vi "TEMPLATE_Regular_Return.vi"(8 "Error In":errorcluster, 11 "LQSerialData In":refnum<class "LQSerialData.lvclass">) -> (0 "Error Out":errorcluster, 2 "Value":string, 3 "LQSerialData Out":refnum<class "LQSerialData.lvclass">)   [LabVIEW 2013, in "Template.lvlib" / "LQSerialData.lvclass"]
uses:
  LQSerialData.lvclass
  LQSerialData.lvclass/LQSerialData.ctl
  LQWidgetEngine/LQWidgetEngine.lvclass
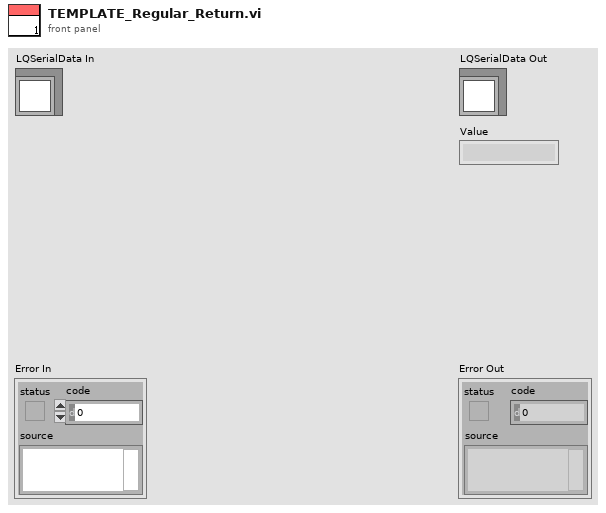
[diagram p1: front panel]
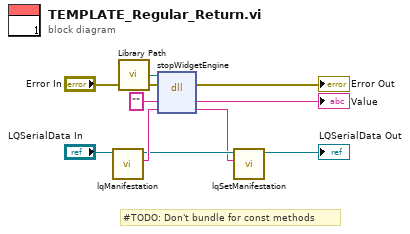
[diagram p0: block diagram]
diagram:
  # "#TODO: Don't bundle for const methods"
  n1 = call "lqManifestation.vi"("LQSerialData in"="LQSerialData In") -> ("Manifestation"=w6:string, "LQSerialData out"=w4:refnum<class "LQSerialData.lvclass">)  [unwired: 9 in]
  n2 = call "Library Path.vi"() -> ("Library Path"=w1:path)
  n3 = dll-call lib="?" fn="stopWidgetEngine"(path in=w1, error in="Error In", "retVal"="", "obj"=w6) -> (error out=→"Error Out":errorcluster, "retVal"=→"Value":string, "obj"=w2:string)  [unwired: 2 in, 1 out]
  n4 = call "lqSetManifestation.vi"("Manifestation"=w2, "LQSerialData in"=w4) -> ("LQSerialData out"=→"LQSerialData Out":refnum<class "LQSerialData.lvclass">)  [unwired: 9 in]
